vi "Init Channel.vi"() -> (3 "Channel Data":T1)   [LabVIEW 2020, in "Flex.lvlib"]
uses:
  Flex.lvlib
  Element.ctl
  Channel Data.ctl
  Element Info.ctl
  Event Data.ctl
  Queue Data.ctl
  Writer Data.ctl
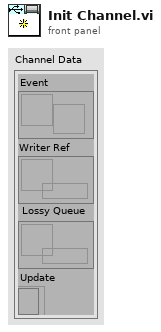
[diagram p1: front panel]
types:
  T1 = typedef "Flex.lvlib/Channel Data.ctl" = cluster{"Event":refnum<user-event>, "Writer Ref":refnum<data-value>, "Lossy Queue":refnum<queue>, "Update":refnum<k4>}
  T2 = typedef "Flex.lvlib/Element Info.ctl" = cluster{"Value":T3, "Updated":timestamp, "Sequence":u32, "Paused":bool}
  T3 = typedef "Flex.lvlib/Element.ctl" = dbl
  T4 = typedef "Flex.lvlib/Writer Data.ctl" = cluster{"Lossless":refnum<queue>[], "Events":bool, "Lossy":bool}
  T5 = typedef "Flex.lvlib/Event Data.ctl" = cluster{"Value":T3, "Closed":bool}
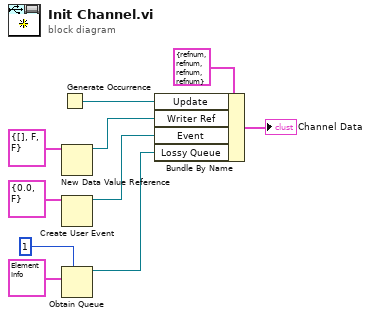
[diagram p0: block diagram]
diagram:
  n1 = Generate Occurrence() -> (w1:refnum<k4>)
  n2 = New Data Value Reference(data value=T4 {"Lossless"=[], "Events"=FALSE, "Lossy"=FALSE} ("Writer Refs")) -> (data value reference=w5:refnum<data-value>)  [unwired: 1 in, 1 out]
  n3 = Create User Event(user event datatype=T5 {"Value"=0.0, "Closed"=FALSE} ("Event Data")) -> (user event=w7:refnum<user-event>)  [unwired: 1 in, 1 out]
  n4 = Obtain Queue(max queue size (-1, unlimited)=1, element data type=T2 {"Value"=0.0, "Updated"=timestamp(0 s since 1904-01-01), "Sequence"=0, "Paused"=FALSE} ("Element Info")) -> (queue out=w2:refnum<queue>)  [unwired: 3 in, 2 out]
  n5 = Bundle By Name(cluster=T1 {"Event"=refnum, "Writer Ref"=refnum, "Lossy Queue"=refnum, "Update"=refnum} ("Channel Data"), "Update"=w1, "Writer Ref"=w5, "Event"=w7, "Lossy Queue"=w2) -> (→"Channel Data":T1)
